vi "LiveVolumeImaging.vi"() -> ()   [LabVIEW 2015]
uses:
  LiveImage_Global.vi
  NIDAQControls/NIDAQGlobals.vi
  NIDAQControls/StateGlobals.vi
  AcquisitionGlobals.vi
panel:
  in  "Set ROI":bool
  out "Max Colors Out":i32[](array[numeric])
  out "XY":T1(plugin-control)
  in  "LUT":T2 {"LUT Red Min" scale=0.0..65535.0; "LUT Red Max" scale=0.8..65535.0; "LUT Green Max" scale=0.8..65535.0}
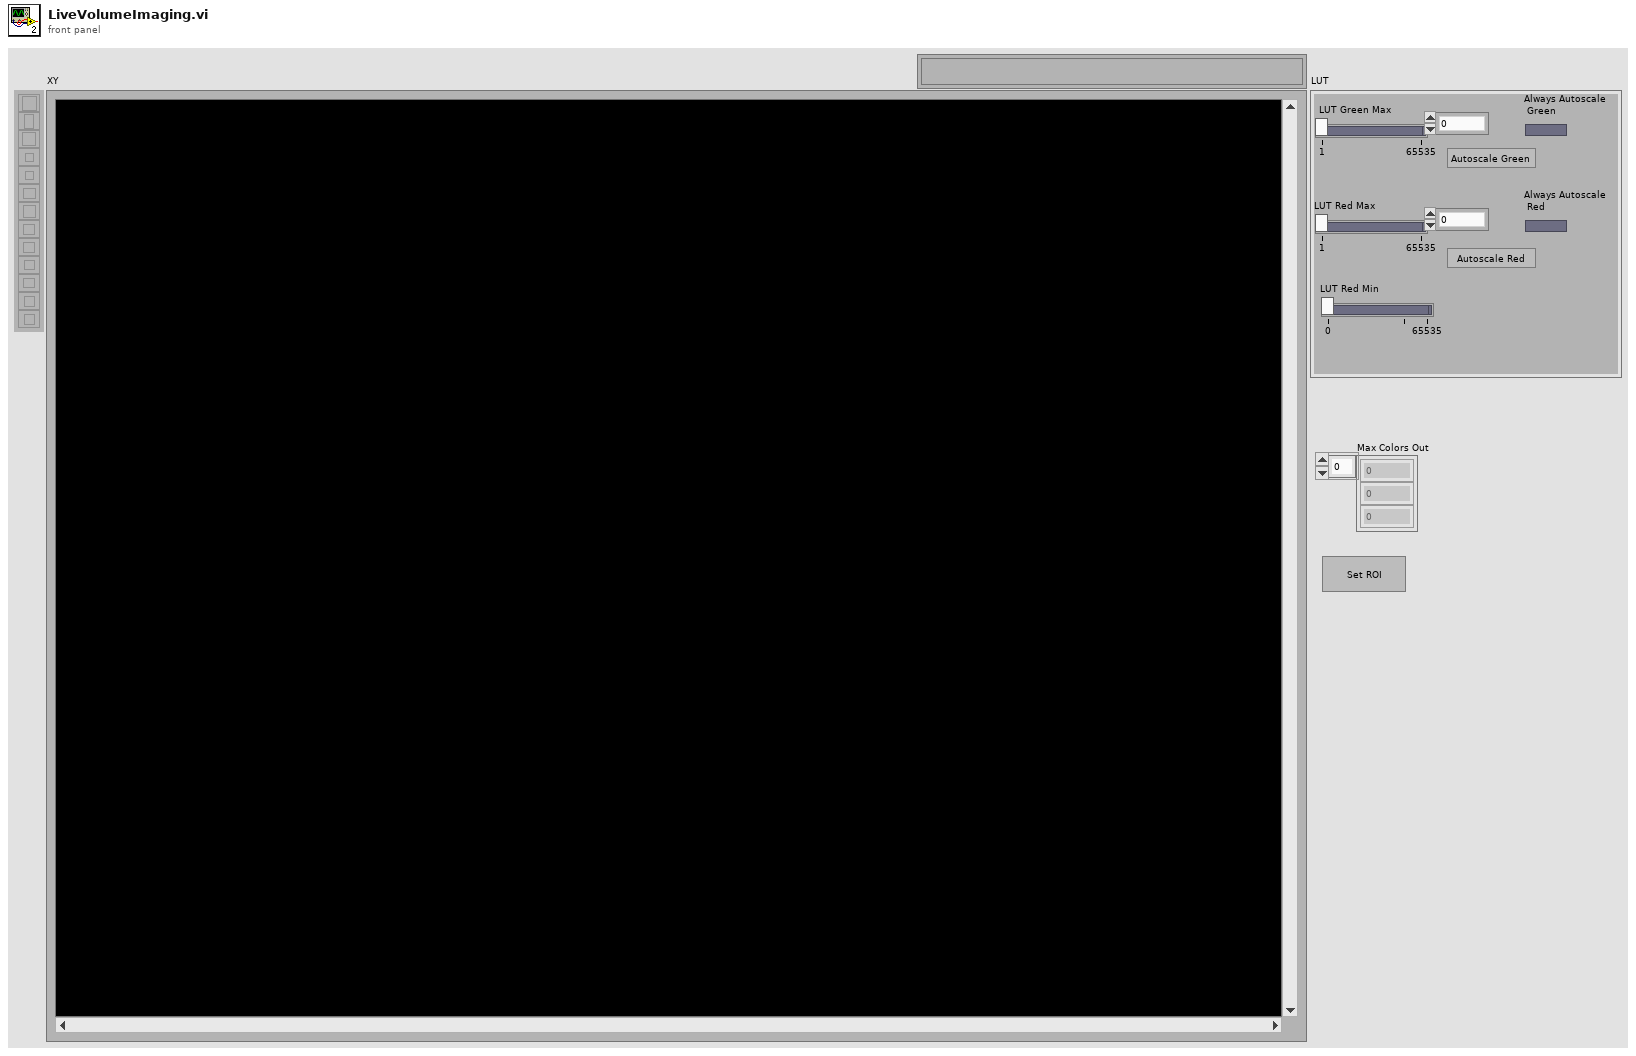
[diagram p1: front panel]
types:
  T1 = typedef "IMAQ Image.ctl" = refnum<image>
  T2 = cluster{"LUT Green Max":u16, "Autoscale Green":bool, "Green LUT Ind":u16, "Always Autoscale\n Green":bool, "LUT Red Max":u16, "Red LUT Ind":u16, "Always Autoscale\n Red":bool, "Autoscale Red":bool, "LUT Red Min":u16}
  T3 = typedef "Image Type" = u32
  T4 = cluster{"Start or New Parameters?":bool, "Laser Mode":string, "Piezo Mode":string, "Begin Or End Acquisition":string, "Acquisition Time":dbl}
  T5 = cluster{"[0]":u16, "[1]":u16, "[2]":u16, "[3]":u16}[][]
  T6 = cluster{"Global Rectangle":i32[], "Contours":cluster{"Contour Type":u32, "ROI Type":u32, "Points":i32[]}[]}
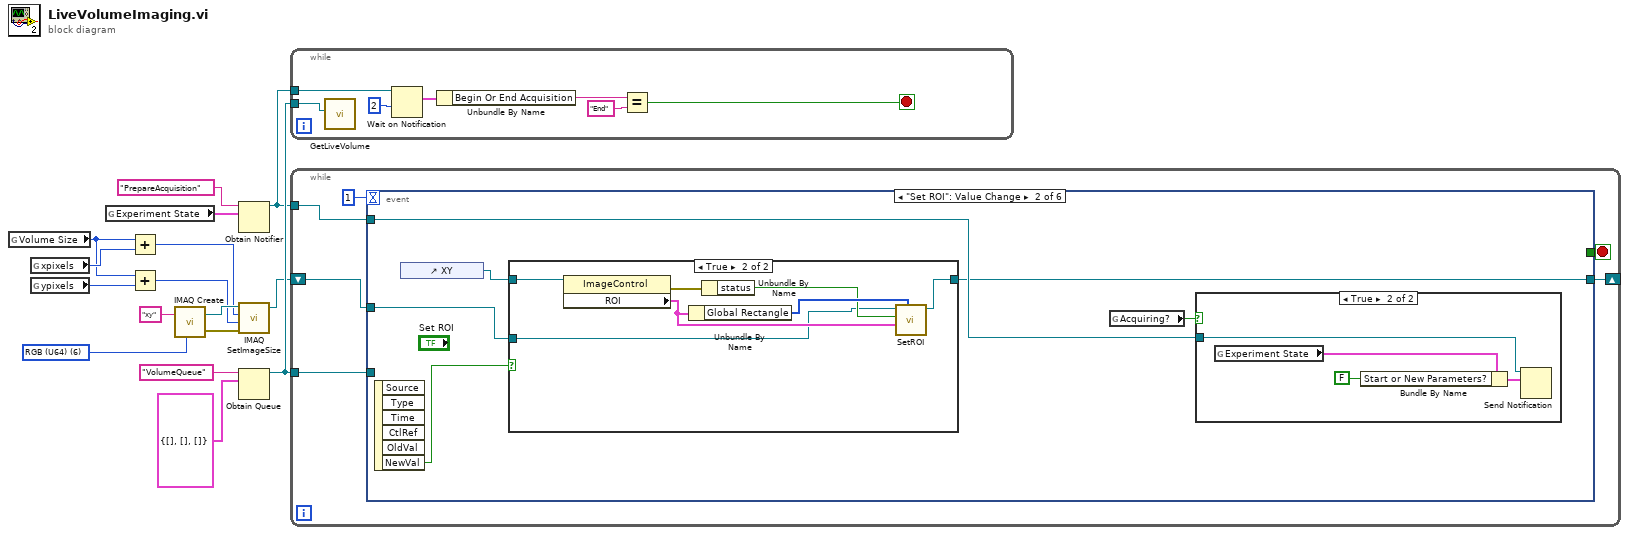
[diagram p0: block diagram]
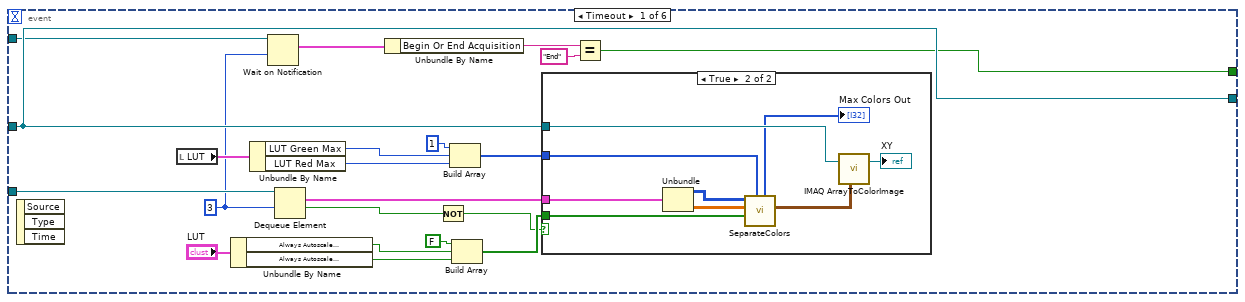
[diagram p2: hidden frame]
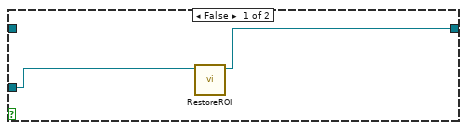
[diagram p5: hidden frame]
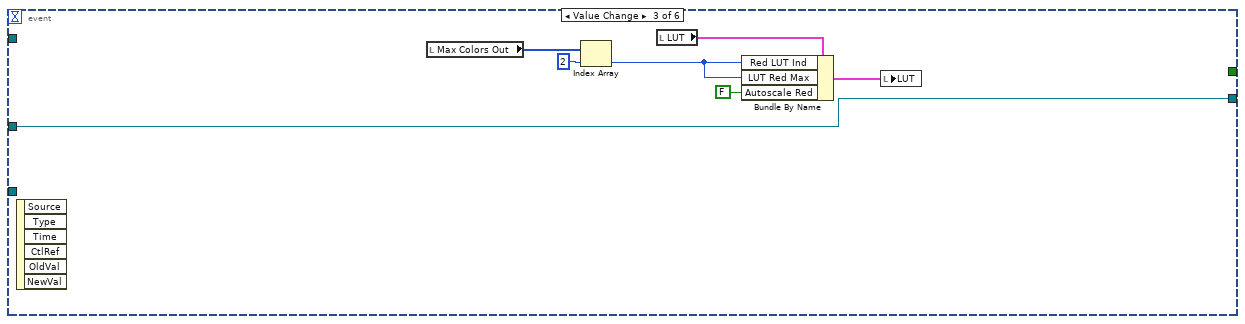
[diagram p6: hidden frame]
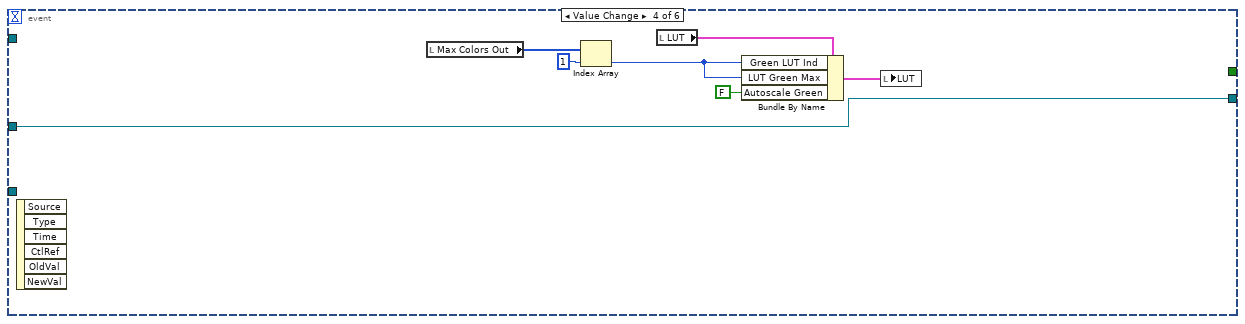
[diagram p7: hidden frame]
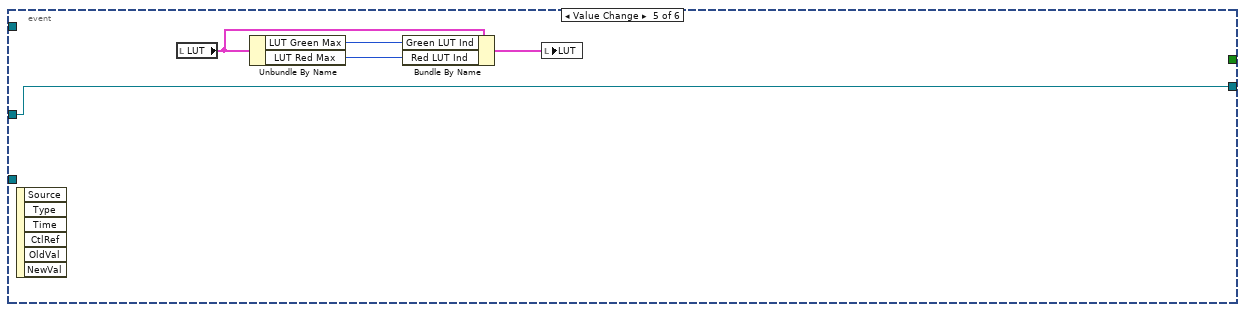
[diagram p8: hidden frame]
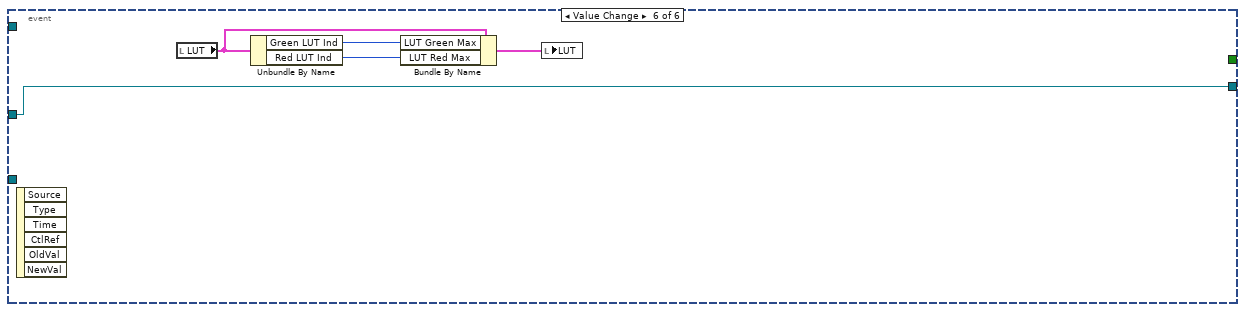
[diagram p9: hidden frame]
diagram:
  w8 = T3 6 items=["Grayscale (U8)", "Grayscale (I16)", "Grayscale (SGL)", "Complex (CSG)", "RGB (U32)", "HSL (U32)", "RGB (U64)", "Grayscale (U16)"] ("Image Type")
  n1 = global read "NIDAQGlobals.vi" "Volume Size"() -> (w2:u16)
  n2 = global read "LiveImage_Global.vi" "xpixels"() -> (w11:i32)
  n3 = global read "LiveImage_Global.vi" "ypixels"() -> (w10:i32)
  n4 = global read "StateGlobals.vi" "Experiment State"() -> (w7:T4)
  n5 = Add(x=w2, y=w11) -> (x+y=w4:i32)
  n6 = Add(x=w2, y=w10) -> (x+y=w3:i32)
  n7 = call "IMAQ Create"("Image Name"="xy", "Image Type"=w8) -> ("New Image"=w12:T1, "error out"=w13:errorcluster)  [unwired: 3 in]
  n8 = Obtain Notifier(name (unnamed)="PrepareAcquisition", notification data type=w7) -> (notifier out=w5:refnum<notifier>)  [unwired: 2 in, 2 out]
  n9 = call "IMAQ SetImageSize"("error in (no error)"=w13, "Y Resolution"=w3, "X Resolution"=w4, "Image"=w12) -> ("Image Out"=w1:T1)  [unwired: 1 in, 1 out]
  n10 = Obtain Queue(name (unnamed)="VolumeQueue", element data type=cluster{u16[][], i32[], dbl[][]} {[], [], []} ("output cluster")) -> (queue out=w15:refnum<queue>)  [unwired: 3 in, 2 out]
  n11 = while {
    tunnel: w15 -> [w23]
    tunnel: w5 -> [w22]
    stop <- w18 stop-if-true
    n12 = call "GetLiveVolume.vi"("VolumeQueueIN"=w23) -> ()  [unwired: 9 in, 2 out]
    n13 = Wait on Notification(notifier=w22, timeout in ms (-1)=2) -> (notification=w21:T4)  [unwired: 2 in, 3 out]
    n14 = Unbundle By Name(w21) -> ("Begin Or End Acquisition"=w20:string)
    n15 = Equal?(x=w20, y="End") -> (x = y?=w18:bool)
  }
  n16 = while {
    tunnel: w15 -> [w29]
    tunnel: w5 -> [w27]
    shift-right: [w24] -> _
    shift-left: w1 -> [w28]
    stop <- w26 stop-if-true
    n17 = event shown="[1] \"Set ROI\": Value Change" {
      selector: _ -> [_ _ _ _ _ _]
      dyn-events: _ -> [_ _ _ _ _ _]
      timeout: 1 -> [_ _ _ _ _ _]
      tunnel: w29 -> [w50 _ _ _ _ _]
      tunnel: w28 -> [w49 w65 w79 w86 w93 w98]
      tunnel: w27 -> [w34 w62 _ _ _ _]
      tunnel: [w31 _ _ _ _ _] -> w26
      tunnel: [w49 w61 w79 w86 w93 w98] -> w24
      event Timeout {
        w35 = 3 ("timeout in ms (-1)")
        n18 = event-data() -> ()  [unwired: 1 in, 3 out]
        n19 = local read "LUT"() -> (w42:T2)
        n20 = Unbundle By Name("LUT") -> ("Always Autoscale\n Green"=w40:bool, "Always Autoscale\n Red"=w41:bool)
        n21 = Unbundle By Name(w42) -> ("LUT Green Max"=w45:u16, "LUT Red Max"=w46:u16)
        n22 = Wait on Notification(notifier=w34, timeout in ms (-1)=w35) -> (notification=w30:T4)  [unwired: 2 in, 3 out]
        n23 = Dequeue Element(queue=w50, timeout in ms (-1)=w35) -> (element=w47:cluster{u16[][], i32[], dbl[][]}, timed out?=w37:bool)  [unwired: 1 in, 2 out]
        n24 = Unbundle By Name(w30) -> ("Begin Or End Acquisition"=w33:string)
        n25 = Not(x=w37) -> (.not. x?=w36:bool)
        n26 = Build Array(u16 1 ("element"), w45, w46) -> (w43:u16[])
        n27 = Build Array(FALSE ("element"), w40, w41) -> (w38:bool[])
        n28 = case shown="True" w36 {
          tunnel: w49 -> [_ w53]
          tunnel: w47 -> [_ w59]
          tunnel: w43 -> [_ w56]
          tunnel: w38 -> [_ w55]
          frame False {
          }
          frame True {
            n29 = Unbundle(w59) -> (w58:u16[][], w57:dbl[][])  [unwired: 1 out]
            n30 = call "SeparateColors.vi"("Max LUT In"=w56, "Autoscale?"=w55, "DAQ Data"=w57, "ImageData"=w58) -> ("Max Projections"=w51:T5, "Max Colors Out"=→"Max Colors Out":i32[])  [unwired: 6 in]
            n31 = call "IMAQ ArrayToColorImage"("Image"=w53, "Image Pixels (U64)"=w51) -> ("Image Out"=→"XY":T1)  [unwired: 3 in, 1 out]
          }
        }
        n32 = Equal?(x=w33, y="End") -> (x = y?=w31:bool)
      }
      event "Set ROI": Value Change {
        n33 = event-data() -> ("NewVal"=w64:bool)  [unwired: 1 in, 5 out]
        n34 = control-ref of="XY"() -> (w60:refnum<vi>)
        n35 = case shown="True" w64 {
          tunnel: w65 -> [w71 w74]
          tunnel: [w70 w73] -> w61
          tunnel: w60 -> [_ w72]
          frame False {
            n36 = call "RestoreROI.vi"("Image In"=w71) -> ("Image Out"=w70:T1)  [unwired: 10 in]
          }
          frame True {
            n37 = property on="Property Node" class="ImageControl"(reference=w72) -> (error out=w78:errorcluster, "ROI"=w77:T6)  [unwired: 1 in, 1 out]
            n38 = Unbundle By Name(w77) -> ("Global Rectangle"=w76:i32[])
            n39 = Unbundle By Name(w78) -> ("status"=w75:bool)
            n40 = call "SetROI.vi"("Global Rectangle"=w76, "ROI In"=w77, "ROI Status"=w75, "Image In"=w74) -> ("Image Out"=w73:T1)  [unwired: 4 in, 3 out]
          }
        }
        n41 = global read "AcquisitionGlobals.vi" "Acquiring?"() -> (w63:bool)
        n42 = case shown="True" w63 {
          tunnel: w62 -> [_ w66]
          frame False {
          }
          frame True {
            n43 = global read "StateGlobals.vi" "Experiment State"() -> (w69:T4)
            n44 = Bundle By Name(cluster=w69, "Start or New Parameters?"=FALSE) -> (w67:T4)
            n45 = Send Notification(notification=w67, notifier=w66) -> ()  [unwired: 1 in, 2 out]
          }
        }
      }
      event "LUT.Autoscale Red": Value Change {
        n46 = event-data() -> ()  [unwired: 1 in, 6 out]
        n47 = local read "Max Colors Out"() -> (w85:i32[])
        n48 = Index Array(array=w85, index=2) -> (element=w82:i32)
        n49 = local read "LUT"() -> (w83:T2)
        n50 = Bundle By Name(cluster=w83, "Red LUT Ind"=w82, "LUT Red Max"=w82, "Autoscale Red"=FALSE) -> (w81:T2)
        n51 = local write "LUT"(w81) -> ()
      }
      event "LUT.Autoscale Green": Value Change {
        n52 = event-data() -> ()  [unwired: 1 in, 6 out]
        n53 = local read "Max Colors Out"() -> (w92:i32[])
        n54 = Index Array(array=w92, index=1) -> (element=w89:i32)
        n55 = local read "LUT"() -> (w90:T2)
        n56 = Bundle By Name(cluster=w90, "Green LUT Ind"=w89, "LUT Green Max"=w89, "Autoscale Green"=FALSE) -> (w88:T2)
        n57 = local write "LUT"(w88) -> ()
      }
      event "LUT.LUT Green Max", "LUT.LUT Red Max": Value Change {
        n58 = event-data() -> ()  [unwired: 1 in, 6 out]
        n59 = local read "LUT"() -> (w97:T2)
        n60 = Unbundle By Name(w97) -> ("LUT Green Max"=w96:u16, "LUT Red Max"=w95:u16)
        n61 = Bundle By Name(cluster=w97, "Green LUT Ind"=w96, "Red LUT Ind"=w95) -> (w94:T2)
        n62 = local write "LUT"(w94) -> ()
      }
      event "LUT.Red LUT Ind", "LUT.Green LUT Ind": Value Change {
        n63 = event-data() -> ()  [unwired: 1 in, 6 out]
        n64 = local read "LUT"() -> (w102:T2)
        n65 = Unbundle By Name(w102) -> ("Green LUT Ind"=w101:u16, "Red LUT Ind"=w100:u16)
        n66 = Bundle By Name(cluster=w102, "LUT Green Max"=w101, "LUT Red Max"=w100) -> (w99:T2)
        n67 = local write "LUT"(w99) -> ()
      }
    }
  }
